vi "S2C_VAR_EditCell.vi"(8 "Error In":errorcluster, 10 "String":string, 11 "CtrlRef":refnum<vi>) -> (0 "Error Out":errorcluster)   [LabVIEW 2015]
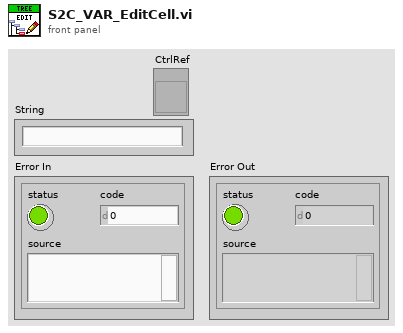
[diagram p1: front panel]
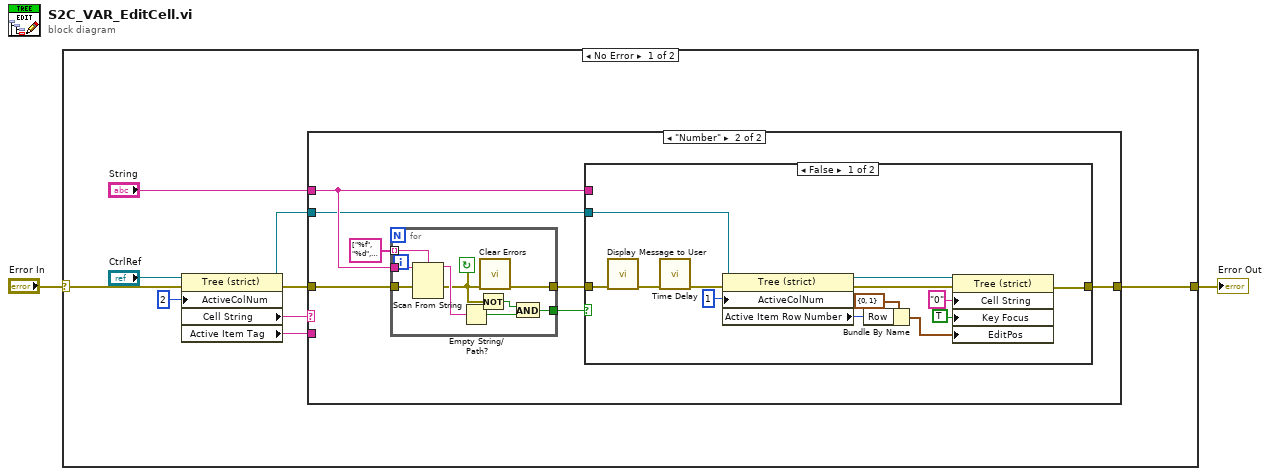
[diagram p0: block diagram]
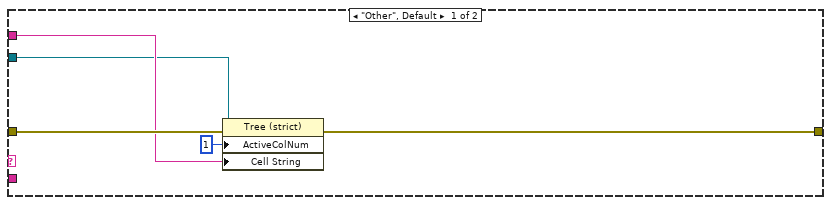
[diagram p2: hidden frame]
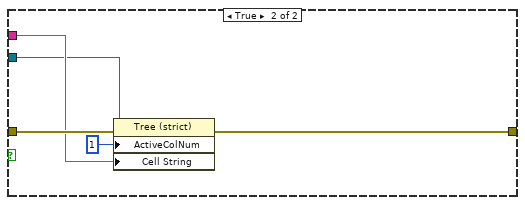
[diagram p3: hidden frame]
diagram:
  n1 = case shown="No Error" "Error In" {
    selector: "Error In" -> [w7 w51]
    tunnel: [w3 w51] -> w1
    frame No Error {
      n2 = property on="Property Node" class="Tree (strict)"(reference="CtrlRef", error in=w7, "ActiveColNum"=2 ("Active Cell:Active Column Number")) -> (reference out=w4:refnum<vi>, error out=w9:errorcluster, "Cell String"=w10:string, "Active Item Tag"=w8:string)
      n3 = case shown="\"Number\"" w10 {
        tunnel: w9 -> [w15 w23]
        tunnel: [w14 w20] -> w3
        tunnel: "String" -> [w13 w19]
        tunnel: w8 -> [_ _]
        tunnel: w4 -> [w12 w17]
        frame "Other", Default {
          n4 = property on="Property Node" class="Tree (strict)"(reference=w12, error in=w15, "ActiveColNum"=1 ("Active Cell:Active Column Number"), "Cell String"=w13) -> (error out=w14:errorcluster)  [unwired: 1 out]
        }
        frame "Number" {
          n5 = for {
            tunnel: w23 -> [w50]
            tunnel: w19 -> [w49]
            tunnel: string[] ["%f", "%d", "%p", "%x", "%o", "%b"] -> [w48] mode=indexing
            tunnel: [w47] -> w21
            tunnel: [w42] -> w18
            stop <- w44 continue-if-true
            n6 = Scan From String(format string=w48, input string=w49, error in=w50) -> (remaining string=w46:string, error out=w44:errorcluster)  [unwired: 3 in, 1 out]
            n7 = Empty String/Path?(string/path=w46) -> (empty?=w45:bool)
            n8 = Not(x=w44) -> (.not. x?=w43:bool)
            n9 = call <vilib>:"Clear Errors.vi"("error in (no error)"=w44) -> ("error out"=w47:errorcluster)  [unwired: 5 in, 1 out]
            n10 = And(x=w43, y=w45) -> (x .and. y?=w42:bool)
          }
          n11 = case shown="False" w18 {
            tunnel: w21 -> [w36 w40]
            tunnel: [w32 w39] -> w20
            tunnel: w19 -> [_ w38]
            tunnel: w17 -> [w25 w37]
            frame False {
              n12 = call "Display Message to User"("error in (no error)"=w36) -> ("error out"=w30:errorcluster)  [unwired: 9 in, 1 out]
              n13 = call "Time Delay"("error in (no error)"=w30) -> ("error out"=w29:errorcluster)  [unwired: 10 in]
              n14 = property on="Property Node" class="Tree (strict)"(reference=w25, error in=w29, "ActiveColNum"=1 ("Active Cell:Active Column Number")) -> (reference out=w24:refnum<vi>, error out=w33:errorcluster, "Active Item Row Number"=w35:i32)
              n15 = Bundle By Name(cluster=cluster{"Row":i32, "Column":i32} {"Row"=0, "Column"=1} ("Edit Position"), "Row"=w35) -> (w26:cluster{"Row":i32, "Column":i32})
              n16 = property on="Property Node" class="Tree (strict)"(reference=w24, error in=w33, "Cell String"="0" ("Active Cell:String"), "Key Focus"=TRUE, "EditPos"=w26) -> (error out=w32:errorcluster)  [unwired: 1 out]
            }
            frame True {
              n17 = property on="Property Node" class="Tree (strict)"(reference=w37, error in=w40, "ActiveColNum"=1 ("Active Cell:Active Column Number"), "Cell String"=w38) -> (error out=w39:errorcluster)  [unwired: 1 out]
            }
          }
        }
      }
    }
    frame Error {
    }
  }
  "Error Out" <- w1
